vi "4p1_HW_Task1_gamagetd.vi"() -> ()   [LabVIEW 2016]
panel:
  out "Actual Height of Fish":dbl
  out "Height of fish through water":dbl
  out "Height fish through glass thickness":dbl
  out "Height fish through air":dbl
  out "Angle of light through water":dbl
  out "Angle light through glass":dbl
  out "Apparent angle person to fish":dbl
  in  "Apparent fish height":dbl
  in  "Refractive Index of Water":dbl
  in  "Refractive Index of Air":dbl
  in  "Refractive Index of glass":dbl
  in  "Distance of fish to glass":dbl
  in  "Thickness of Glass":dbl
  in  "Distance of person to wall":dbl
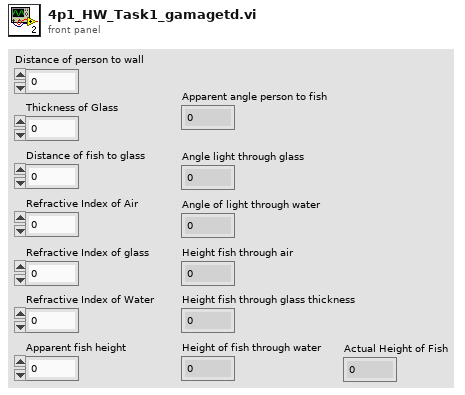
[diagram p1: front panel]
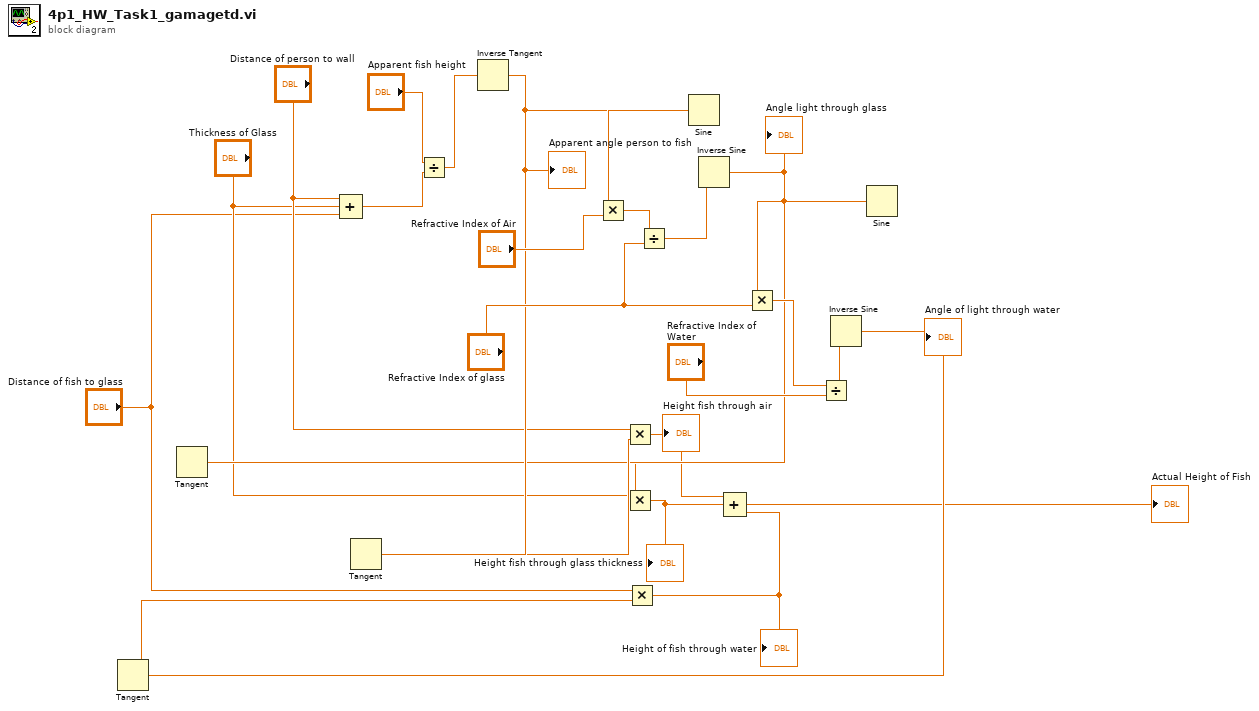
[diagram p0: block diagram]
diagram:
  n1 = Compound Arithmetic op=ADD("Distance of person to wall", "Thickness of Glass", "Distance of fish to glass") -> (w25:dbl)
  n2 = Divide(x="Apparent fish height", y=w25) -> (x/y=w23:dbl)
  n3 = Inverse Tangent(1:w23) -> (0:w13:dbl)
  "Apparent angle person to fish" <- w13
  n4 = Tangent(1:w13) -> (0:w12:dbl)
  n5 = Multiply(x="Distance of person to wall", y=w12) -> (x*y=w4:dbl)
  "Height fish through air" <- w4
  n6 = Sine(x=w13) -> (sin(x)=w20:dbl)
  n7 = Multiply(x=w20, y="Refractive Index of Air") -> (x*y=w19:dbl)
  n8 = Divide(x=w19, y="Refractive Index of glass") -> (x/y=w21:dbl)
  n9 = Inverse Sine(1:w21) -> (0:w10:dbl)
  "Angle light through glass" <- w10
  n10 = Tangent(1:w10) -> (0:w9:dbl)
  n11 = Multiply(x="Thickness of Glass", y=w9) -> (x*y=w3:dbl)
  "Height fish through glass thickness" <- w3
  n12 = Sine(x=w10) -> (sin(x)=w18:dbl)
  n13 = Multiply(x=w18, y="Refractive Index of glass") -> (x*y=w16:dbl)
  n14 = Divide(x=w16, y="Refractive Index of Water") -> (x/y=w14:dbl)
  n15 = Inverse Sine(1:w14) -> (0:w6:dbl)
  "Angle of light through water" <- w6
  n16 = Tangent(1:w6) -> (0:w7:dbl)
  n17 = Multiply(x="Distance of fish to glass", y=w7) -> (x*y=w2:dbl)
  "Height of fish through water" <- w2
  n18 = Compound Arithmetic op=ADD(w4, w3, w2) -> (→"Actual Height of Fish":dbl)
